vi "geis.vi"(0 "IP adress":string="192.109.209.229", 1 "stop":bool, 2 "Channel":u8(ring) items=["1", "2", "3", "4", "5", "6", "7", "8", "9", "10", "11", "12", "13", "14", "15", "16"], 3 "GEIS Parameters":T2={"Step_number"=0, "Initial_Current_step"=0.0, "vs_initial "=TRUE, "Final_Current_step"=0.001, "vs_final"=TRUE, "Duration_step"=1.0, "Record_every_dE"=0.1, "Record_every_dT"=0.1, "Initial_frequency"=100000.0, "sweep"=FALSE, "Final_frequency"=1.0, "Frequency_number"=51, "Amplitude_Current"=0.001, "Wait_for_steady"=2.0, "Average_N_times"=1, "Correction"=TRUE, "I_Range"=7, "Bandwidth"=5, "em"=1, "ce"=0} {"ce" items=["Standard", "CE to ground"]; "em" max=10 format="%.5f"; "Initial_Current_step" min=-10 max=10 format="%.5f"; "Step_number" min=0 step=1; "I_Range" items=["1pA", "1nA", "10nA", "100nA", "1µA", "10µA", "100µA", "1mA", "10mA", "100mA", "1A", "Booster"]; "Bandwidth" items=["1"=1, "2"=2, "3"=3, "4"=4, "5"=5, "6"=6, "7"=7, "8"=8, "9"=9]; "Wait_for_steady" min=0 format="%.2f"; "Record_every_dT" min=0 format="%.2e"; "Record_every_dE" min=0 format="%.2e"; "Duration_step" min=0 format="%.5f"; "Final_Current_step" min=-10 max=10 format="%.5f"; "Average_N_times" min=1 max=1000 step=1; "Amplitude_Current" min=0 max=100 format="%.2e"; "Final_frequency" min=1e-05 max=1000000 format="%.2e"; "Frequency_number" min=1 max=10000; "Initial_frequency" min=1e-05 max=1000000 format="%.2e"}, 4 "Exit":bool, 5 "Start":bool, 8 "Draw":T1(ring)) -> (6 "Number of points":i32=52, 7 "XY Graph":cluster{"Data p1":sgl[], "Data p1":dbl[]}[](graph))   [LabVIEW 2014]
doc: "The Staircase Galvano Electrochemical Impedance Spectroscopy (SGEIS) technique is close to the SPEIS technique, except that the current is controlled instead of the potential.\n\nIn general, in this VI, the first thing to do is to start by establishing the connection with the instrument defined by its IP adress, then load the firmware in the channel selected, get the information on the plugged channels, load protocol on a channel, start/stop the protocol, retreive data and draw the graph.\nThis technique is applied just for channels with impedance capabilities (Zboard)."
uses:
  LLB/dll_Functions.llb/GEISParameters.ctl
panel:
  in  "Display Parameters?":bool caption="Display Parameters"
  out "DllPath":path caption="DLL Path"
  out "LibVersion":string caption="DLL Version"
  out "Data P0":sgl[][](array[numeric])=[[4.8e-05, 1.2033013, 0.0012545494], [7.2e-05, 4.099232, 0.0030298461], [9.6e-05, 5.4905596, 0.0034574724], [0.00040800002, 5.594096, 0.0031739129], [0.00086400006, 5.697314, 0.00286901], [0.0014160001, 5.800989, 0.0025610582], [0.002112, 5.903515, 0.002253106], [0.0030480002, 6.0050545, 0.0019497279], [0.0045120004, 6.105221, 0.0016379646], [0.008280001, 6.2053866, 0.0013155299], [0.100008, 6.222552, 0.0012118629], [0.200016, 6.223086, 0.0012103383], [0.300024, 6.223086, 0.0012126251], [0.400032, 6.2233143, 0.0012133875], [0.50004, 6.2231617, 0.0012141496], [0.600048, 6.2229333, 0.0012133875], [0.700056, 6.2229333, 0.0012103383], [0.800064, 6.2227044, 0.0012095761], [0.90007204, 6.2233143, 0.0012149118]]
  out "Data P1":sgl[][](array[numeric])=[[99999.99, 0.015896028, 2.4134535e-05, -0.31541085, 6.2027836, 0.0012093844, 0.0, 0.028001478, 2.4202996e-05, -0.21167731, -6.8013325, -0.001209385, 0.0, 1.296, 8.0], [79789.055, 0.020694803, 3.145496e-05, -0.31517792, 6.1967587, 0.0012085777, 0.0, 0.036134787, 3.1510877e-05, -0.20527963, -6.7949142, -0.0012085784, 0.0, 1.584, 8.0], [63671.867, 0.027115118, 3.95239e-05, -0.36039186, 6.1889963, 0.0012069115, 0.0, 0.04638151, 3.95688e-05, -0.23149349, -6.7864842, -0.0012069122, 0.0, 1.872, 8.0], [50804.684, 0.035882276, 4.949095e-05, -0.40444195, 6.178996, 0.0012048192, 0.0, 0.05973892, 4.952679e-05, -0.25926352, -6.77554, -0.0012048199, 0.0, 2.16, 8.0], [40539.06, 0.048188828, 6.136454e-05, -0.4440093, 6.1657524, 0.0012020994, 0.0, 0.077702746, 6.139315e-05, -0.28762102, -6.7610307, -0.0012021001, 0.0, 2.448, 8.0], [32343.752, 0.06770085, 7.88223e-05, -0.47251844, 6.1465006, 0.0011982684, 0.0, 0.10554845, 7.884587e-05, -0.31181583, -6.739913, -0.0011982691, 0.0, 2.736, 8.0], [25812.496, 0.12644306, 0.0001329111, -0.48514298, 6.0997047, 0.0011887155, 0.0, 0.19051811, 0.00013293685, -0.32698154, -6.6886125, -0.0011887162, 0.0, 3.024, 8.0], [20593.748, 0.23297587, 0.00022114319, -0.47706103, 6.015843, 0.0011718888, 0.0, 0.34030145, 0.00022117054, -0.3275948, -6.596549, -0.0011718895, 0.0, 3.312, 8.0], [16429.69, 0.37617812, 0.00032387703, -0.45101714, 5.8985395, 0.0011485365, 0.0, 0.5348972, 0.00032390282, -0.31515712, -6.4677424, -0.0011485372, 0.0, 3.6000001, 8.0], [13109.373, 0.55603534, 0.00044012873, -0.4103434, 5.7451816, 0.0011180385, 0.0, 0.7737537, 0.00044015126, -0.2906543, -6.299325, -0.0011180392, 0.0, 3.888, 8.0], [10460.936, 0.7749276, 0.00057313335, -0.36184657, 5.5526934, 0.001079828, 0.0, 1.0605142, 0.0005731519, -0.25886726, -6.0878835, -0.0010798287, 1.0, 4.176, 8.0], [8351.5625, 1.0352163, 0.00072714745, -0.31150156, 5.3164287, 0.0010371187, 1.0, 1.3994575, 0.0007271621, -0.22451091, -5.8299828, -0.0010371194, 1.0, 4.609, 8.0], [6660.1553, 1.3410046, 0.000907536, -0.26282227, 5.0436444, 0.0009789959, 1.0, 1.7970788, 0.00090754736, -0.19028175, -5.5293727, -0.0009789965, 2.0, 4.947, 8.0], [5313.953, 1.5113798, 0.0009967732, -0.21961367, 4.8940244, 0.0009556693, 1.0, 2.0129824, 0.000996781, -0.15885389, -5.3671427, -0.00095566985, 2.0, 5.57, 8.0], [4241.786, 1.5454612, 0.0010015898, -0.18297291, 4.878454, 0.0009537674, 1.0, 2.0500069, 0.0010015944, -0.13264023, -5.3505425, -0.0009537679, 2.0, 6.213, 8.0], [3385.4163, 1.5790181, 0.0010115571, -0.153041, 4.8648095, 0.00095176516, 1.0, 2.0889149, 0.0010115607, -0.111195564, -5.3358197, -0.0009517657, 2.0, 6.857, 8.0], [2699.3184, 1.5802759, 0.0010046018, -0.1293776, 4.883166, 0.0009544167, 1.0, 2.0867875, 0.0010046042, -0.09421384, -5.3556128, -0.0009544172, 2.0, 7.501, 8.0], [2153.4448, 1.5856456, 0.001002952, -0.11168504, 4.8972144, 0.0009564839, 1.0, 2.0912726, 0.0010029528, -0.08150327, -5.370766, -0.0009564844, 2.0, 8.1449995, 8.0], [1717.748, 1.5895984, 0.0010019304, -0.09921706, 4.9112163, 0.0009589054, 1.0, 2.0948448, 0.0010019315, -0.072561264, -5.38597, -0.0009589059, 2.0, 8.792, 8.0], [1372.1951, 1.5920151, 0.0010009218, -0.09178877, 4.924607, 0.0009613617, 1.0, 2.0966747, 0.0010009219, -0.06731814, -5.400561, -0.0009613622, 2.0, 9.439, 8.0], [1096.7545, 1.6009942, 0.0010047532, -0.08871567, 4.9333324, 0.000961253, 1.0, 2.1073825, 0.001004754, -0.06525302, -5.4094787, -0.00096125354, 2.0, 9.871, 8.0], [871.93097, 1.5816059, 0.0009906995, -0.09027839, 4.959241, 0.000966918, 1.0, 2.0806665, 0.0009906992, -0.06663093, -5.4381466, -0.00096691854, 2.0, 10.307, 8.0], [696.1138, 1.5729876, 0.0009832102, -0.09623489, 4.9737277, 0.0009698118, 1.0, 2.0679011, 0.0009832109, -0.07122159, -5.454079, -0.0009698124, 2.0, 10.741, 8.0], [555.8894, 1.6019666, 0.0009985057, -0.106960624, 4.9539285, 0.00096688373, 1.0, 2.1039863, 0.0009985064, -0.07941079, -5.4326506, -0.0009668843, 2.0, 11.394, 8.0], [443.43906, 1.6082691, 0.0009985616, -0.122988224, 4.9526095, 0.0009666943, 1.0, 2.1093283, 0.000998562, -0.091551304, -5.4311996, -0.00096669485, 2.0, 12.053, 8.0], [353.75473, 1.6163155, 0.0009975499, -0.14474046, 4.9489985, 0.00096599624, 1.0, 2.1154938, 0.0009975497, -0.10804355, -5.427236, -0.0009659968, 2.0, 12.715, 8.0], [281.8943, 1.6319947, 0.000997945, -0.1731171, 4.939253, 0.000964064, 1.0, 2.1291127, 0.0009979454, -0.12966967, -5.416549, -0.00096406456, 2.0, 13.377, 8.0], [225.3606, 1.6545873, 0.000997958, -0.20826769, 4.9249706, 0.00096138736, 1.0, 2.1484613, 0.0009979575, -0.15665877, -5.4009104, -0.0009613879, 2.0, 14.045, 8.0], [180.28844, 1.6867937, 0.0009969639, -0.25068158, 4.9050946, 0.0009575135, 1.0, 2.1753373, 0.0009969644, -0.18979812, -5.3791265, -0.0009575141, 2.0, 14.722, 8.0], [143.75787, 1.7397344, 0.0009973684, -0.30079174, 4.872224, 0.00095120573, 1.0, 2.2215395, 0.0009973678, -0.22964483, -5.3430943, -0.0009512063, 2.0, 15.411, 8.0], [114.59661, 1.8171204, 0.0009974693, -0.3567279, 4.8248806, 0.00094198145, 1.0, 2.2893379, 0.0009974696, -0.27555776, -5.2911463, -0.00094198197, 2.0, 16.109, 8.0], [91.552734, 1.9272654, 0.0009971086, -0.4146781, 4.7582307, 0.00092904264, 2.0, 2.3872557, 0.0009971082, -0.32522857, -5.217652, -0.00092904316, 2.0, 17.039999, 8.0], [72.87778, 2.0835702, 0.0009966118, -0.47080094, 4.6631265, 0.00091063714, 2.0, 2.5288415, 0.0009966121, -0.37639964, -5.1133604, -0.00091063767, 2.0, 17.782999, 8.0], [58.30223, 2.290216, 0.0009965424, -0.5163753, 4.536835, 0.00088618894, 2.0, 2.7210877, 0.000996542, -0.42156878, -4.9748783, -0.00088618946, 2.0, 18.546999, 8.0], [46.50297, 2.5567615, 0.0009965401, -0.54690737, 4.373813, 0.0008546952, 2.0, 2.9750876, 0.0009965405, -0.45663965, -4.796084, -0.00085469574, 2.0, 19.302, 8.0], [36.95101, 2.8818939, 0.0009962525, -0.55650496, 4.17603, 0.0008164121, 2.0, 3.292113, 0.0009962524, -0.47500235, -4.5792, -0.00081641256, 2.0, 20.077, 8.0], [29.592804, 3.234223, 0.0009962742, -0.5438912, 3.963954, 0.0007754039, 2.0, 3.6432135, 0.000996275, -0.47317147, -4.346668, -0.0007754044, 2.0, 20.93, 8.0], [23.588463, 3.6068342, 0.0009961284, -0.5106709, 3.7440598, 0.0007329593, 2.0, 4.0214486, 0.0009961289, -0.45162058, -4.1054997, -0.0007329597, 2.0, 21.862, 8.0], [18.780045, 3.9640598, 0.0009960186, -0.46161065, 3.5391219, 0.00069332117, 2.0, 4.3898535, 0.0009960192, -0.41360545, -3.8807545, -0.0006933216, 2.0, 22.863, 8.0], [15.024037, 4.271375, 0.0009959555, -0.40523124, 3.3689148, 0.00066039263, 2.0, 4.710784, 0.0009959557, -0.36663783, -3.694098, -0.00066039304, 2.0, 23.906, 8.0], [11.982363, 4.520932, 0.0009950611, -0.3458606, 3.2371411, 0.0006348915, 2.0, 4.9737754, 0.000995061, -0.31517577, -3.5495536, -0.0006348918, 2.0, 24.949, 8.0], [9.574144, 2.38077, 0.0005031747, -0.28917873, 4.6680098, 0.0009119648, 2.0, 2.6153588, 0.0005031747, -0.26482016, -5.1187296, -0.00091196527, 2.0, 25.382, 8.0], [7.6293964, 2.4353614, 0.0004999304, -0.23806715, 4.644746, 0.0009074361, 2.0, 2.6731777, 0.00049993006, -0.21878657, -5.0931625, -0.0009074366, 2.0, 25.922, 8.0], [6.084501, 2.4750657, 0.00049832056, -0.19374752, 4.6285977, 0.0009043441, 2.0, 2.7155764, 0.0004983205, -0.17844573, -5.075479, -0.0009043446, 2.0, 26.594, 8.0], [4.858519, 2.5030587, 0.0004974475, -0.15684187, 4.617654, 0.0009022134, 2.0, 2.7455964, 0.0004974477, -0.14467418, -5.0634913, -0.000902214, 2.0, 27.432001, 8.0], [3.8752477, 2.52257, 0.0004969658, -0.12630916, 4.6102643, 0.0009008552, 2.0, 2.7666035, 0.00049696607, -0.11720729, -5.055331, -0.00090085575, 2.0, 28.479, 8.0], [3.1001983, 2.5355425, 0.0004967685, -0.101694584, 4.6055255, 0.0008999815, 2.0, 2.7805579, 0.0004967687, -0.09457946, -5.050148, -0.000899982, 2.0, 29.784, 8.0], [2.4660668, 2.5443485, 0.00049676636, -0.0811795, 4.602378, 0.0008993778, 2.0, 2.7900364, 0.00049676653, -0.075683355, -5.046685, -0.0008993783, 2.0, 31.421001, 8.0], [1.9649143, 2.550054, 0.0004967066, -0.06482482, 4.600377, 0.0008989733, 2.0, 2.7961702, 0.0004967067, -0.060593843, -5.0444574, -0.00089897384, 2.0, 33.471, 8.0], [1.5725644, 2.5537558, 0.0004967495, -0.051944494, 4.599086, 0.00089873036, 2.0, 2.8001752, 0.0004967496, -0.04870844, -5.043045, -0.0008987309, 2.0, 36.029, 8.0], [1.2520034, 2.5562146, 0.00049671344, -0.04138118, 4.5982056, 0.00089857634, 2.0, 2.8028417, 0.00049671356, -0.03896928, -5.042108, -0.00089857687, 2.0, 39.239, 8.0], [1.0016024, 2.557709, 0.00049671053, -0.03315392, 4.597694, 0.0008984848, 2.0, 2.8044465, 0.00049671077, -0.031377077, -5.0415564, -0.00089848536, 2.0, 43.248, 8.0]]
  out "Exit 2":bool=TRUE
  # "Instructions:\nBefore running the VI you must type a valid IP adress that corresponds to the instrument.Then press the Run button to execute this VI.\nWhile this VI is running, choose the available channel, enter the SGEIS parameters or keep the default\n values, then press the button start to begin the experience. \nChoose the waveform to draw : Nyquist, modZ, theta...\nPress the stop button to end experience and the exit button to stop the VI execution."
  # "Set I (A)  vs. previous"
  # "Before EIS  stay for ts (s)"
  # "and record every dE (V)"
  # "or every dt (s)"
  # "Start EIS from  Fi (Hz)"
  # "sweep linear/logarithmic"
  # "to Ff (Hz)"
  # "for Nf frequencies"
  # "with the amplitude (A)"
  # "wait for Pw"
  # "average Na times"
  # "drift correction"
  # "with I Range"
  # "bandwidth"
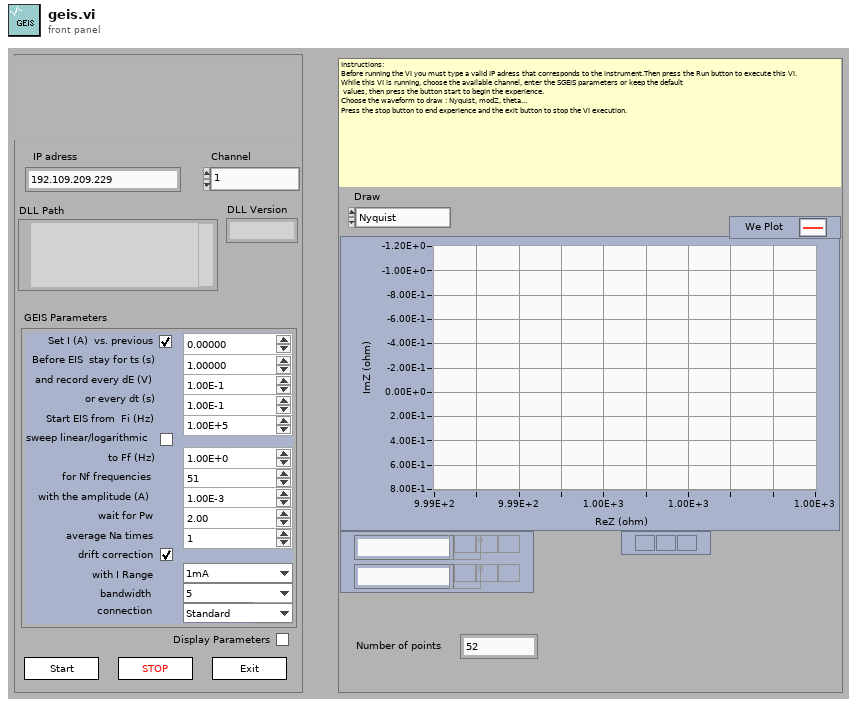
[diagram p1: front panel]
types:
  T1 = enum16{"Nyquist", "modZ", "theta", "modE", "modI", "Edc", "Idc", "E range", "I range", "f(t)"}
  T2 = typedef "GEISParameters.ctl" = cluster{"Step_number":i32, "Initial_Current_step":sgl, "vs_initial ":bool, "Final_Current_step":sgl, "vs_final":bool, "Duration_step":sgl, "Record_every_dE":sgl, "Record_every_dT":sgl, "Initial_frequency":sgl, "sweep":bool, "Final_frequency":sgl, "Frequency_number":i32, "Amplitude_Current":sgl, "Wait_for_steady":sgl, "Average_N_times":i32, "Correction":bool, "I_Range":u16, "Bandwidth":u16, "em":u16, "ce":u16}
  T3 = cluster{"LibVersion":string, "StringLength":u32, "DllPath":path}
  T4 = cluster{"Channel":i32, "BoardVersion":i32, "BoardSerialCode":i32, "FirmwareCode":i32, "FirmwareVersion":i32, "XilinxVersion":i32, "AmpCode":i32, "NbAmp":i32, "LcBoard":i32, "Zboard":i32, "MuxBoard":i32, "GPRAboard":i32, "MemSize":i32, "MemFilled":i32, "state":i32, "MaxIRange":i32, "MinIRange":i32, "MaxBandwidth":i32, "NbOfTechniques":i32}
  T5 = typedef "TechniqueParameters.ctl" = cluster{"String Label":string, "Type":i32, "Valeur":i32, "Index":i32}
  T6 = cluster{"string before end tag":string, i32, i32, i32}[]
  T7 = cluster{"IRQskipped":i32, "NbRaws":i32, "NbCols":i32, "Technique Index":i32, "TechniqueID":i32, "PrcessIndex":i32, "loop":i32, "StartTime":dbl, "MuxPad":i32}
  T8 = cluster{"State":i32, "MemFilled":i32, "TimeBase":sgl, " Ewe":sgl, " EweRangeMin":sgl, " EweRangeMax":sgl, "Ece":sgl, "EceRangeMin":sgl, "EceRangeMax":sgl, "Eoverflow":i32, "I":sgl, "IRange":i32, "Ioverflow":i32, "ElapsedTime":sgl, "Freq":sgl, "Rcomp":sgl, "Saturation":sgl, "OptErr":i32, "OptPos":i32}
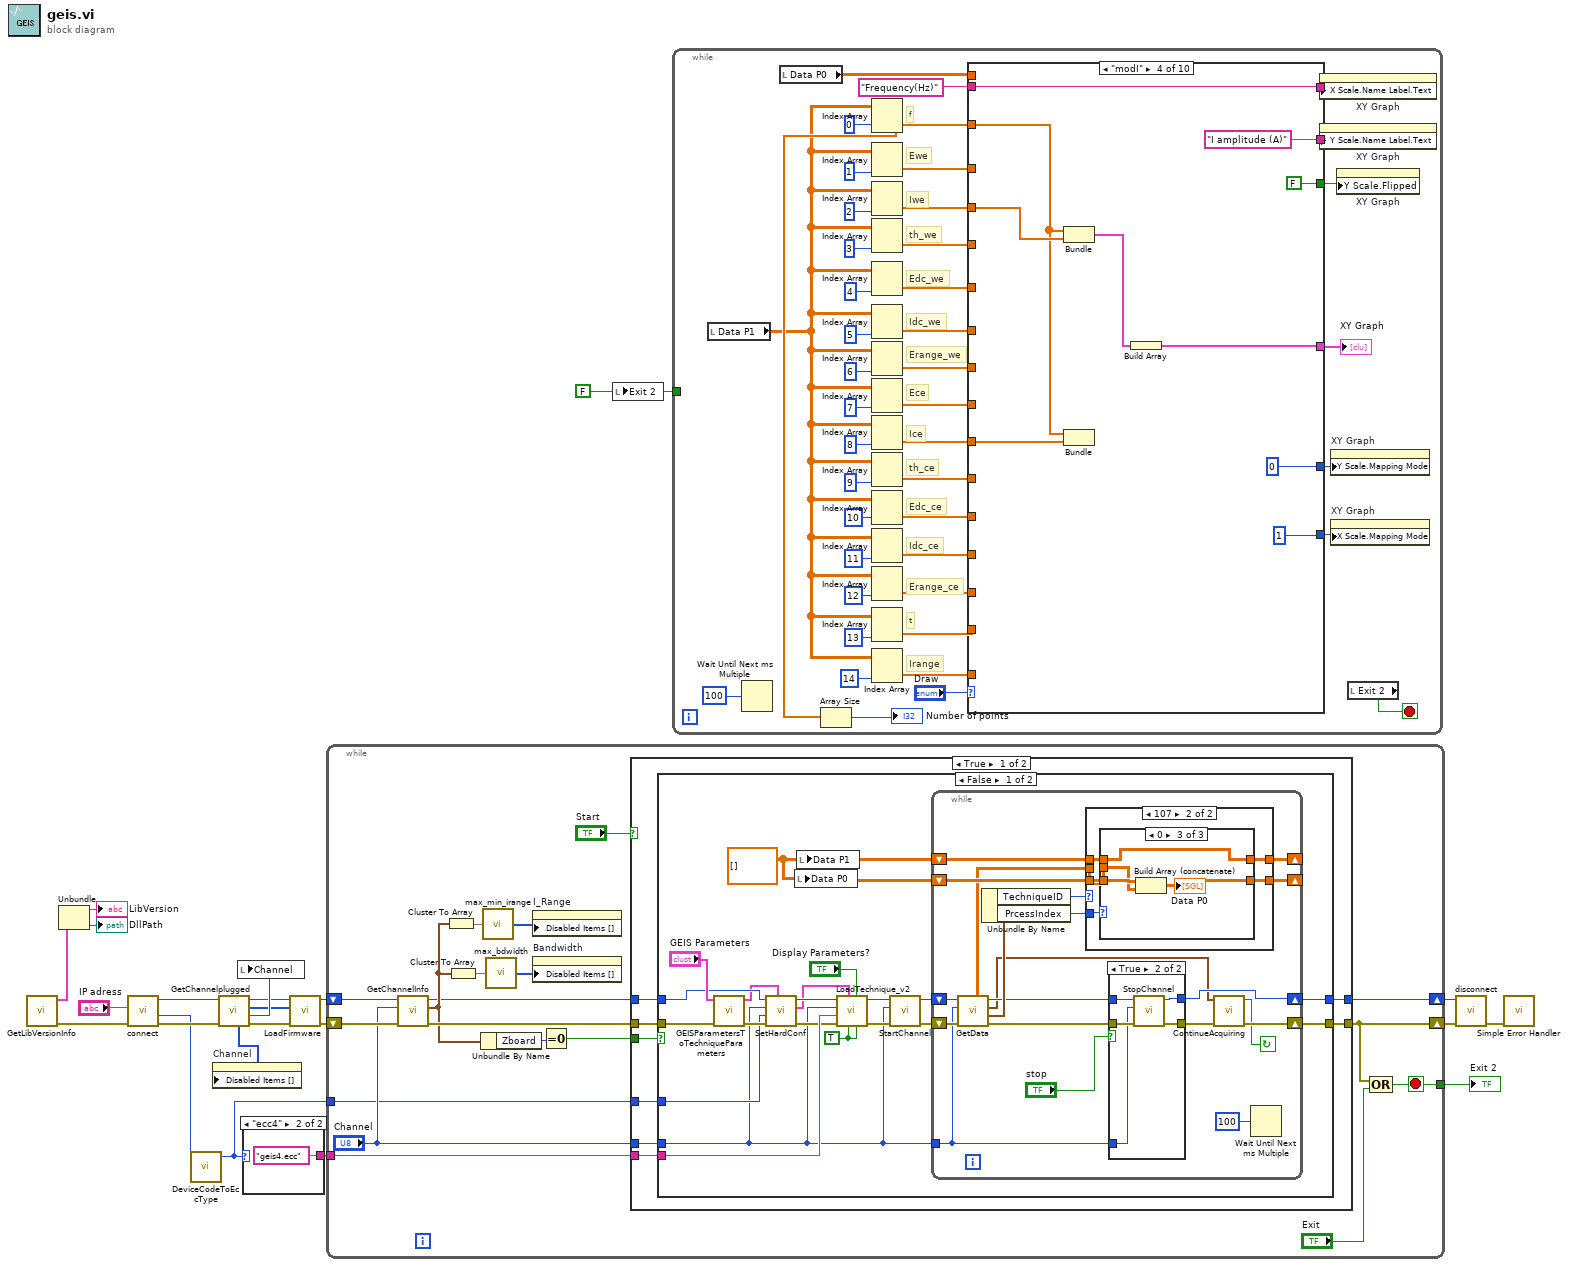
[diagram p0: block diagram]
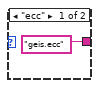
[diagram p2: hidden frame]
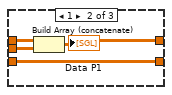
[diagram p5: hidden frame]
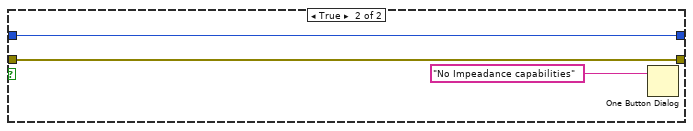
[diagram p7: hidden frame]
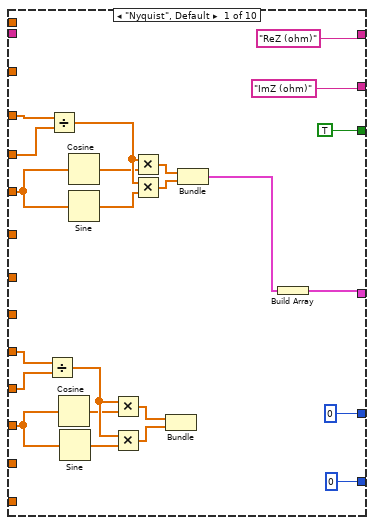
[diagram p9: hidden frame]
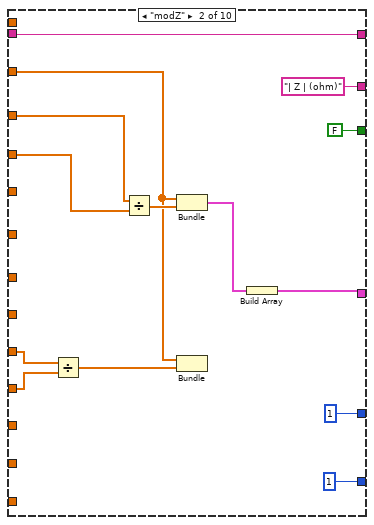
[diagram p10: hidden frame]
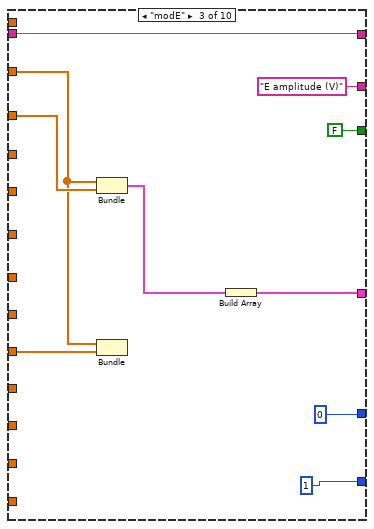
[diagram p11: hidden frame]
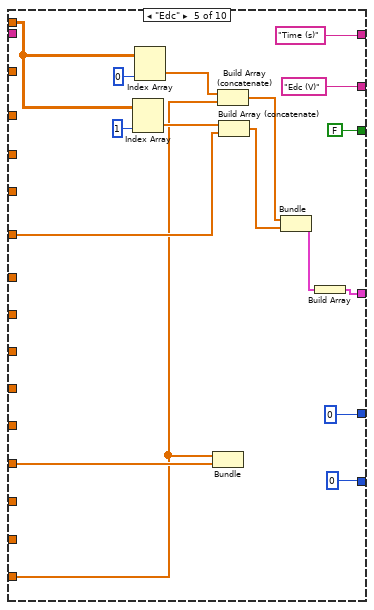
[diagram p12: hidden frame]
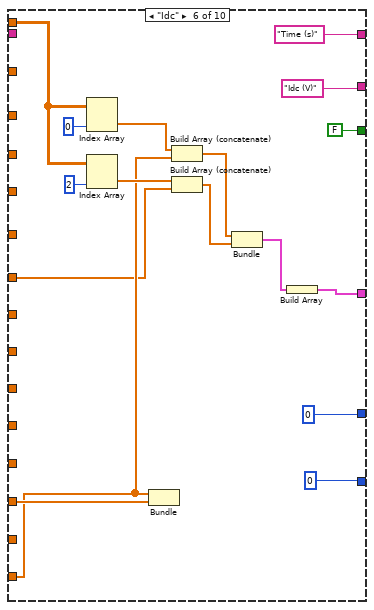
[diagram p13: hidden frame]
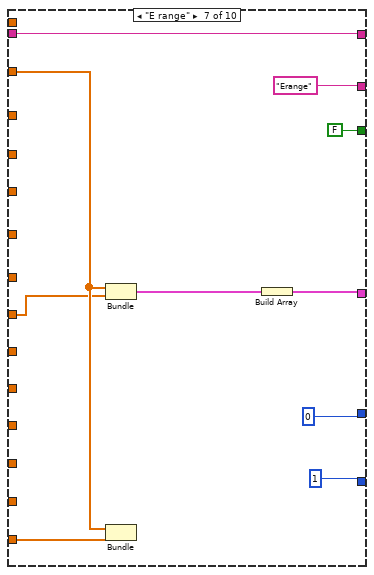
[diagram p14: hidden frame]
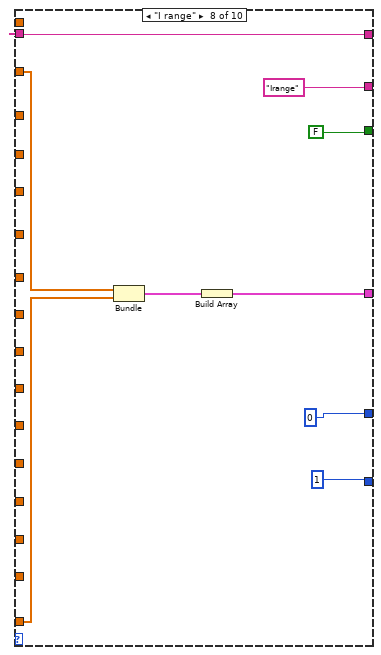
[diagram p15: hidden frame]
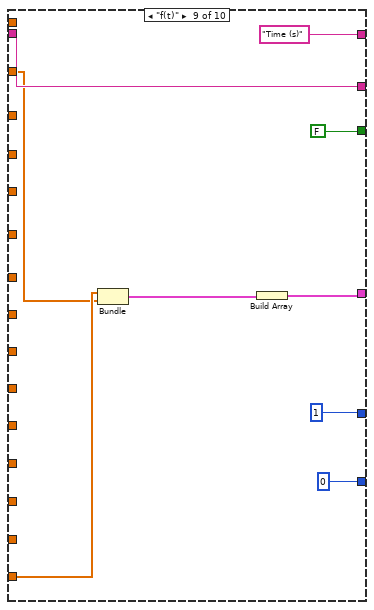
[diagram p16: hidden frame]
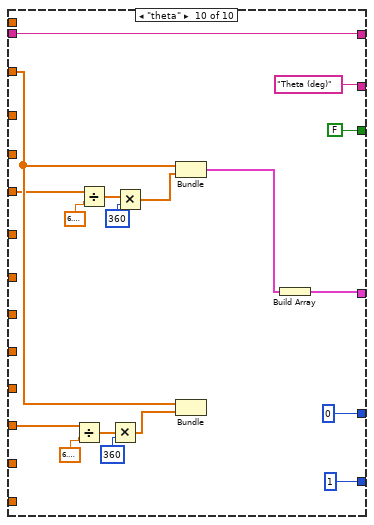
[diagram p17: hidden frame]
diagram:
  w20 = FALSE
  n1 = call "GetLibVersionInfo.vi"() -> ("error out"=w1:errorcluster, "LibInfo"=w4:T3)  [unwired: 10 in]
  n2 = Unbundle(w4) -> ("LibVersion"=→"LibVersion":string, "DllPath"=→"DllPath":path)  [unwired: 1 out]
  n3 = call "connect.vi"("error in (no error)"=w1, "IP"="IP adress") -> ("error out"=w16:errorcluster, "Device Code"=w8:i32, "ID Out"=w18:i32)  [unwired: 6 in, 1 out]
  n4 = call "DeviceCodeToEccType.vi"("Device Code"=w8) -> ("EccType"=w5:enum16{"ecc", "ecc4"})  [unwired: 4 in]
  n5 = call "GetChannelplugged.vi"("error in (no error)"=w16, "ID In"=w18) -> ("error out"=w15:errorcluster, "FirstPluggedChannel"=w21:u8, "PluggedChannels"=w10:u8[], "ID Out"=w13:i32, "DisabledChannels"=w11:i32[])  [unwired: 5 in]
  n6 = property on="Channel" class="Ring (strict)"("Disabled Items []"=w11) -> ()  [unwired: 2 in, 2 out]
  n7 = local write "Channel"(w21) -> ()
  n8 = case shown="\"ecc4\"" w5 {
    tunnel: ["geis.ecc" ("FName") "geis4.ecc" ("FName")] -> w7
    frame "ecc" {
    }
    frame "ecc4" {
    }
  }
  n9 = call "LoadFirmware.vi"("error in (no error)"=w15, "Channels"=w10, "ID In"=w13) -> ("error out"=w14:errorcluster, "ID Out"=w12:i32)  [unwired: 6 in, 1 out]
  n10 = while {
    shift-right: [w28] -> w9
    shift-left: w14 -> [w35]
    tunnel: [w26] -> w19
    shift-right: [w38] -> w17
    shift-left: w12 -> [w31]
    tunnel: w7 -> [w29]
    tunnel: w5 -> [w25]
    stop <- w26 stop-if-true
    n11 = call "GetChannelInfo.vi"("error in (no error)"=w35, "Channel"="Channel", "ID"=w31) -> ("error out"=w33:errorcluster, "Channel information"=w32:T4, "ID Out"=w30:i32)  [unwired: 6 in]
    n12 = Cluster To Array(cluster=w32) -> (array=w40:i32[])
    n13 = Cluster To Array(cluster=w32) -> (array=w39:i32[])
    n14 = Unbundle By Name(w32) -> ("Zboard"=w42:i32)
    n15 = call "max_min_irange.vi"("resources"=w40) -> ("disabled ranges"=w36:i32[])
    n16 = call "max_bdwidth.vi"("resources"=w39) -> ("disabled ranges"=w37:i32[])
    n17 = property on="I_Range" class="Ring (strict)"("Disabled Items []"=w36) -> ()  [unwired: 2 in, 2 out]
    n18 = property on="Bandwidth" class="Ring (strict)"("Disabled Items []"=w37) -> ()  [unwired: 2 in, 2 out]
    n19 = Equal To 0?(x=w42) -> (x = 0?=w41:bool)
    n20 = case shown="True" "Start" {
      tunnel: "Channel" -> [w50 _]
      tunnel: [w51 w121] -> w28
      tunnel: w33 -> [w49 w121]
      tunnel: w41 -> [w48 _]
      tunnel: w30 -> [w47 w120]
      tunnel: [w46 w120] -> w38
      tunnel: w29 -> [w45 _]
      tunnel: w25 -> [w44 _]
      frame True {
        n21 = case shown="False" w48 {
          tunnel: [w71 w118] -> w51
          tunnel: w50 -> [w53 _]
          tunnel: w49 -> [w67 w118]
          tunnel: w47 -> [w57 w117]
          tunnel: [w61 w117] -> w46
          tunnel: w45 -> [w63 _]
          tunnel: w44 -> [w54 _]
          frame False {
            w66 = TRUE ("First Protocol")
            w70 = sgl[][] [] ("Data")
            n22 = call "GEISParametersToTechniqueParameters.vi"("error in (no error)"=w67, "GEIS Parameters"="GEIS Parameters") -> ("error out"=w60:errorcluster, "TechniqueParameters"=w56:T5[])  [unwired: 8 in]
            n23 = call "SetHardConf.vi"("Params Values"=w56, "error in (no error)"=w60, "EccType"=w54, "Channel"=w53, "ID In"=w57) -> ("error out"=w59:errorcluster, "Params Values Trimed"=w55:T6, "ID Out"=w58:i32)  [unwired: 4 in]
            n24 = local write "Data P0"(w70) -> ()
            n25 = local write "Data P1"(w70) -> ()
            n26 = call "LoadTechnique_v2.vi"("Last Protocol"=w66, "Display Parameters?"="Display Parameters?", "First Protocol"=w66, "TechniqueParameters"=w55, "error in (no error)"=w59, "FName"=w63, "Selected Channel"=w53, "ID In"=w58) -> ("error out"=w64:errorcluster, "ID  Out"=w65:i32)  [unwired: 2 in]
            n27 = call "StartChannel.vi"("error in (no error)"=w64, "Channel"=w53, "ID In"=w65) -> ("error out"=w68:errorcluster, "ID Out"=w62:i32)  [unwired: 7 in]
            n28 = while {
              shift-right: [w77] -> w71
              shift-left: w68 -> [w90]
              shift-right: [w86] -> _
              shift-left: w70 -> [w87]
              shift-right: [w84] -> _
              shift-left: w70 -> [w85]
              shift-right: [w74] -> w61
              shift-left: w62 -> [w79]
              tunnel: w53 -> [w72]
              stop <- w75 continue-if-true
              n29 = call "GetData.vi"("error in (no error)"=w90, "Channel"=w72, "ID In"=w79) -> ("error out"=w88:errorcluster, "Data information"=w91:T7, "Current values"=w73:T8, "ID Out"=w78:i32, "Data"=w80:dbl[][])  [unwired: 4 in]
              n30 = Unbundle By Name(w91) -> ("TechniqueID"=w82:i32, "PrcessIndex"=w81:i32)
              n31 = case shown="107" w82 {
                tunnel: w87 -> [w93 w99]
                tunnel: [w93 w98] -> w86
                tunnel: w85 -> [w92 w97]
                tunnel: [w92 w96] -> w84
                tunnel: w80 -> [_ w95]
                tunnel: w81 -> [_ w94]
                frame Default {
                }
                frame 107 {
                  n32 = case shown="0" w94 {
                    tunnel: [w101 w103 w106] -> w98
                    tunnel: w99 -> [w101 w104 w106]
                    tunnel: [w100 w102 w107] -> w96
                    tunnel: w97 -> [w100 w102 w109]
                    tunnel: w95 -> [_ w105 w108]
                    frame Default {
                    }
                    frame 1 {
                      n33 = Build Array (concatenate)(w104, w105) -> (w103:dbl[][])
                      "Data P1" <- w103
                    }
                    frame 0 {
                      n34 = Build Array (concatenate)(w109, w108) -> (w107:dbl[][])
                      "Data P0" <- w107
                    }
                  }
                }
              }
              n35 = case shown="True" "stop" {
                tunnel: [w111 w116] -> w76
                tunnel: w88 -> [w111 w115]
                tunnel: w78 -> [w110 w114]
                tunnel: [w110 w113] -> w74
                tunnel: w72 -> [_ w112]
                frame False {
                }
                frame True {
                  n36 = call "StopChannel.vi"("error in (no error)"=w115, "Channel"=w112, "ID In"=w114) -> ("error out"=w116:errorcluster, "ID Out"=w113:i32)  [unwired: 7 in]
                }
              }
              n37 = call "ContinueAcquiring.vi"("error in"=w76, "Current values"=w73) -> ("error out"=w77:errorcluster, "ContinueAcquiring?"=w75:bool)  [unwired: 8 in]
              n38 = Wait Until Next ms Multiple(millisecond multiple=u32 100) -> ()  [unwired: 1 out]
            }
          }
          frame True {
            n39 = One Button Dialog(message="No Impeadance capabilities" ("error source (\" \")")) -> ()  [unwired: 1 in, 1 out]
          }
        }
      }
      frame False {
      }
    }
    n40 = Compound Arithmetic op=OR(w28, "Exit") -> (w26:bool)
  }
  "Exit 2" <- w19
  n41 = local write "Exit 2"(w20) -> ()
  n42 = while {
    tunnel: w20 -> [_]
    stop <- w153 stop-if-true
    # "Erange_ce"
    # "Idc_ce"
    # "Edc_ce"
    # "th_ce"
    # "Ice"
    # "Ece"
    # "t"
    # "Irange"
    # "Erange_we"
    # "Idc_we"
    # "Edc_we"
    # "th_we"
    # "Iwe"
    # "Ewe"
    # "f"
    n43 = local read "Data P1"() -> (w123:sgl[][])
    n44 = Wait Until Next ms Multiple(millisecond multiple=u32 100) -> ()  [unwired: 1 out]
    n45 = local read "Data P0"() -> (w122:sgl[][])
    n46 = Index Array(array=w123, index (col)=0 ("Index")) -> (element=w137:sgl[])  [unwired: 1 in]
    n47 = Array Size(array=w137) -> (size(s)=→"Number of points":i32)
    n48 = Index Array(array=w123, index (col)=1 ("Index")) -> (element=w138:sgl[])  [unwired: 1 in]
    n49 = Index Array(array=w123, index (col)=2 ("Index")) -> (element=w143:sgl[])  [unwired: 1 in]
    n50 = Index Array(array=w123, index (col)=3 ("Index")) -> (element=w158:sgl[])  [unwired: 1 in]
    n51 = Index Array(array=w123, index (col)=4 ("disabled index (col)")) -> (element=w152:sgl[])  [unwired: 1 in]
    n52 = Index Array(array=w123, index (col)=5 ("disabled index (col)")) -> (element=w149:sgl[])  [unwired: 1 in]
    n53 = Index Array(array=w123, index (col)=6 ("index (row)")) -> (element=w139:sgl[])  [unwired: 1 in]
    n54 = Index Array(array=w123, index (col)=7) -> (element=w130:sgl[])  [unwired: 1 in]
    n55 = Index Array(array=w123, index (col)=8) -> (element=w129:sgl[])  [unwired: 1 in]
    n56 = Index Array(array=w123, index (col)=9) -> (element=w128:sgl[])  [unwired: 1 in]
    n57 = Index Array(array=w123, index (col)=10) -> (element=w127:sgl[])  [unwired: 1 in]
    n58 = Index Array(array=w123, index (col)=11) -> (element=w126:sgl[])  [unwired: 1 in]
    n59 = Index Array(array=w123, index (col)=12) -> (element=w125:sgl[])  [unwired: 1 in]
    n60 = Index Array(array=w123, index (col)=13 ("disabled index (col)")) -> (element=w140:sgl[])  [unwired: 1 in]
    n61 = Index Array(array=w123, index (col)=14 ("disabled index (col)")) -> (element=w141:sgl[])  [unwired: 1 in]
    n62 = case shown="\"modI\"" "Draw" {
      tunnel: w137 -> [_ w194 w204 w215 _ _ w260 w268 w277 w288]
      tunnel: w138 -> [w170 w192 w211 _ _ _ _ _ _ _]
      tunnel: w143 -> [w169 w191 _ w221 _ _ _ _ _ _]
      tunnel: ["ImZ (ohm)" ("Y Scale.Name Label.Text") "| Z | (ohm)" ("Y Scale.Name Label.Text") "E amplitude (V)" ("Y Scale.Name Label.Text") "I amplitude (A)" ("Y Scale.Name Label.Text") "Edc (V)" ("Y Scale.Name Label.Text") "Idc (V)" ("Y Scale.Name Label.Text") "Erange" ("Y Scale.Name Label.Text") "Irange" ("Y Scale.Name Label.Text") w282 "Theta (deg)" ("Y Scale.Name Label.Text")] -> w160
      tunnel: w158 -> [w165 _ _ _ _ _ _ _ _ w286]
      tunnel: ["ReZ (ohm)" ("Y Scale.Name Label.Text") w199 w209 w219 "Time (s)" ("Y Scale.Name Label.Text") "Time (s)" ("Y Scale.Name Label.Text") w265 w274 "Time (s)" ("Y Scale.Name Label.Text") w301] -> w157
      tunnel: "Frequency(Hz)" ("Y Scale.Name Label.Text") -> [_ w199 w209 w219 _ _ w265 w274 w282 w301]
      tunnel: [TRUE ("Y Scale.Flipped") FALSE ("Y Scale.Flipped") FALSE ("Y Scale.Flipped") FALSE ("Y Scale.Flipped") FALSE ("Y Scale.Flipped") FALSE ("Y Scale.Flipped") FALSE ("Y Scale.Flipped") FALSE FALSE FALSE ("Y Scale.Flipped")] -> w155
      tunnel: [u8 0 ("X Scale.Mapping Mode") u8 1 ("X Scale.Mapping Mode") u8 1 ("X Scale.Mapping Mode") u8 1 ("X Scale.Mapping Mode") 0 0 1 1 0 u8 1 ("X Scale.Mapping Mode")] -> w154
      tunnel: w152 -> [_ _ _ _ w226 _ _ _ _ _]
      tunnel: w149 -> [_ _ _ _ _ w240 _ _ _ _]
      tunnel: w139 -> [_ _ _ _ _ _ w257 _ _ _]
      tunnel: w141 -> [_ _ _ _ _ _ _ w269 _ _]
      tunnel: w140 -> [_ _ _ _ w223 w241 _ _ w278 _]
      tunnel: [0 1 u8 0 ("X Scale.Mapping Mode") u8 0 ("X Scale.Mapping Mode") 0 0 0 0 1 0 ("X Scale.Mapping Mode")] -> w145
      tunnel: w130 -> [w168 w190 w205 _ _ _ _ _ _ _]
      tunnel: w129 -> [w167 w189 _ w214 _ _ _ _ _ _]
      tunnel: w128 -> [w166 _ _ _ _ _ _ _ _ w285]
      tunnel: w127 -> [_ _ _ _ w225 _ _ _ _ _]
      tunnel: w126 -> [_ _ _ _ _ w242 _ _ _ _]
      tunnel: w125 -> [_ _ _ _ _ _ w258 _ _ _]
      tunnel: [w175 w188 w202 w212 w224 w243 w256 w266 w275 w284] -> w124
      tunnel: w122 -> [_ _ _ _ w227 w244 _ _ _ _]
      frame "Nyquist", Default {
        n63 = Divide(x=w168, y=w167) -> (x/y=w172:sgl[])
        n64 = Divide(x=w170, y=w169) -> (x/y=w174:sgl[])
        n65 = Cosine(x=w166) -> (cos(x)=w171:sgl[])
        n66 = Sine(x=w166) -> (sin(x)=w177:sgl[])
        n67 = Cosine(x=w165) -> (cos(x)=w173:sgl[])
        n68 = Sine(x=w165) -> (sin(x)=w187:sgl[])
        n69 = Multiply(x=w172, y=w171) -> (x*y=w179:sgl[])
        n70 = Multiply(x=w172, y=w177) -> (x*y=w178:sgl[])
        n71 = Multiply(x=w174, y=w173) -> (x*y=w181:sgl[])
        n72 = Multiply(x=w174, y=w187) -> (x*y=w182:sgl[])
        n73 = Bundle(w179, w178) -> ()  [unwired: 1 in, 1 out]
        n74 = Bundle(w181, w182) -> (w176:cluster{sgl[], sgl[]})  [unwired: 1 in]
        n75 = Build Array(w176) -> (w175:cluster{sgl[], sgl[]}[])
      }
      frame "modZ" {
        n76 = Divide(x=w190, y=w189) -> (x/y=w195:sgl[])
        n77 = Divide(x=w192, y=w191) -> (x/y=w201:sgl[])
        n78 = Bundle("Data P1"=w194, w201) -> (w193:cluster{"Data P1":sgl[], sgl[]})  [unwired: 1 in]
        n79 = Bundle("Data P1"=w194, w195) -> ()  [unwired: 1 in, 1 out]
        n80 = Build Array(w193) -> (w188:cluster{"Data P1":sgl[], sgl[]}[])
      }
      frame "modE" {
        n81 = Bundle("Data P1"=w204, "Data P1"=w211) -> (w203:cluster{"Data P1":sgl[], "Data P1":sgl[]})  [unwired: 1 in]
        n82 = Bundle("Data P1"=w204, "Data P1"=w205) -> ()  [unwired: 1 in, 1 out]
        n83 = Build Array(w203) -> (w202:cluster{"Data P1":sgl[], "Data P1":sgl[]}[])
      }
      frame "modI" {
        n84 = Bundle("Data P1"=w215, "Data P1"=w221) -> (w213:cluster{"Data P1":sgl[], "Data P1":sgl[]})  [unwired: 1 in]
        n85 = Bundle("Data P1"=w215, "Data P1"=w214) -> ()  [unwired: 1 in, 1 out]
        n86 = Build Array(w213) -> (w212:cluster{"Data P1":sgl[], "Data P1":sgl[]}[])
      }
      frame "Edc" {
        n87 = Index Array(array=w227, index (col)=1 ("Index")) -> (element=w228:sgl[])  [unwired: 1 in]
        n88 = Index Array(array=w227, index (col)=0 ("Index")) -> (element=w229:sgl[])  [unwired: 1 in]
        n89 = Bundle("Data P1"=w223, "Data P1"=w225) -> ()  [unwired: 1 in, 1 out]
        n90 = Build Array (concatenate)(w229, w223) -> (w233:sgl[])
        n91 = Build Array (concatenate)(w228, w226) -> (w232:sgl[])
        n92 = Bundle(w233, w232) -> (w230:cluster{sgl[], sgl[]})  [unwired: 1 in]
        n93 = Build Array(w230) -> (w224:cluster{sgl[], sgl[]}[])
      }
      frame "Idc" {
        n94 = Index Array(array=w244, index (col)=0 ("Index")) -> (element=w248:sgl[])  [unwired: 1 in]
        n95 = Index Array(array=w244, index (col)=2 ("Index")) -> (element=w247:sgl[])  [unwired: 1 in]
        n96 = Bundle("Data P1"=w241, "Data P1"=w242) -> ()  [unwired: 1 in, 1 out]
        n97 = Build Array (concatenate)(w248, w241) -> (w246:sgl[])
        n98 = Build Array (concatenate)(w247, w240) -> (w245:sgl[])
        n99 = Bundle(w246, w245) -> (w251:cluster{sgl[], sgl[]})  [unwired: 1 in]
        n100 = Build Array(w251) -> (w243:cluster{sgl[], sgl[]}[])
      }
      frame "E range" {
        n101 = Bundle("Data P1"=w260, "Data P1"=w257) -> (w259:cluster{"Data P1":sgl[], "Data P1":sgl[]})  [unwired: 1 in]
        n102 = Bundle("Data P1"=w260, "Data P1"=w258) -> ()  [unwired: 1 in, 1 out]
        n103 = Build Array(w259) -> (w256:cluster{"Data P1":sgl[], "Data P1":sgl[]}[])
      }
      frame "I range" {
        n104 = Bundle("Data P1"=w268, "Data P1"=w269) -> (w267:cluster{"Data P1":sgl[], "Data P1":sgl[]})  [unwired: 1 in]
        n105 = Build Array(w267) -> (w266:cluster{"Data P1":sgl[], "Data P1":sgl[]}[])
      }
      frame "f(t)" {
        n106 = Bundle("Data P1"=w278, "Data P1"=w277) -> (w276:cluster{"Data P1":sgl[], "Data P1":sgl[]})  [unwired: 1 in]
        n107 = Build Array(w276) -> (w275:cluster{"Data P1":sgl[], "Data P1":sgl[]}[])
      }
      frame "theta" {
        n108 = Divide(x=w285, y=6.283185307179586) -> (x/y=w290:dbl[])
        n109 = Divide(x=w286, y=6.283185307179586) -> (x/y=w298:dbl[])
        n110 = Multiply(x=w290, y=360) -> (x*y=w292:dbl[])
        n111 = Multiply(x=w298, y=360) -> (x*y=w295:dbl[])
        n112 = Bundle("Data P1"=w288, w295) -> (w287:cluster{"Data P1":sgl[], dbl[]})  [unwired: 1 in]
        n113 = Bundle("Data P1"=w288, w292) -> ()  [unwired: 1 in, 1 out]
        n114 = Build Array(w287) -> (w284:cluster{"Data P1":sgl[], dbl[]}[])
      }
    }
    "XY Graph" <- w124
    n115 = property on="XY Graph" class="XYGraph (strict)"("X Scale.Name Label.Text"=w157) -> ()  [unwired: 2 in, 2 out]
    n116 = property on="XY Graph" class="XYGraph (strict)"("Y Scale.Name Label.Text"=w160) -> ()  [unwired: 2 in, 2 out]
    n117 = property on="XY Graph" class="XYGraph (strict)"("Y Scale.Mapping Mode"=w145) -> ()  [unwired: 2 in, 2 out]
    n118 = property on="XY Graph" class="XYGraph (strict)"("X Scale.Mapping Mode"=w154) -> ()  [unwired: 2 in, 2 out]
    n119 = property on="XY Graph" class="XYGraph (strict)"("Y Scale.Flipped"=w155) -> ()  [unwired: 2 in, 2 out]
    n120 = local read "Exit 2"() -> (w153:bool)
  }
  n121 = call "disconnect.vi"("error in (no error)"=w9, "ID In"=w17) -> ("error out"=w6:errorcluster)  [unwired: 9 in]
  n122 = call <vilib>:"Simple Error Handler.vi"("error in (no error)"=w6) -> ()  [unwired: 4 in, 5 out]
